vi "Load_from_Project.vi"(8 "error in (no error)":errorcluster, 9 "index":string, 10 "buildObject":T1, 11 "IB_RegData in":refnum<class "IB_RegData.lvclass">) -> (0 "error out":errorcluster, 1 "index out":string, 2 "buildObject out":T1, 3 "IB_RegData out":refnum<class "IB_RegData.lvclass">)   [LabVIEW 2020, in "IB_RegData.lvclass"]
uses:
  <vilib>/AppBuilder/IB_Classes/RegData/IB_RegData.lvclass
  <vilib>/AppBuilder/IB_Classes/RegData/IB_RegData.lvclass/IB_RegData.ctl
  <vilib>/AppBuilder/IB_RW_Project/IB_RW_Project_PropBag_Action.ctl
  <resource>/Framework/Providers/API/ItemRef.ctl
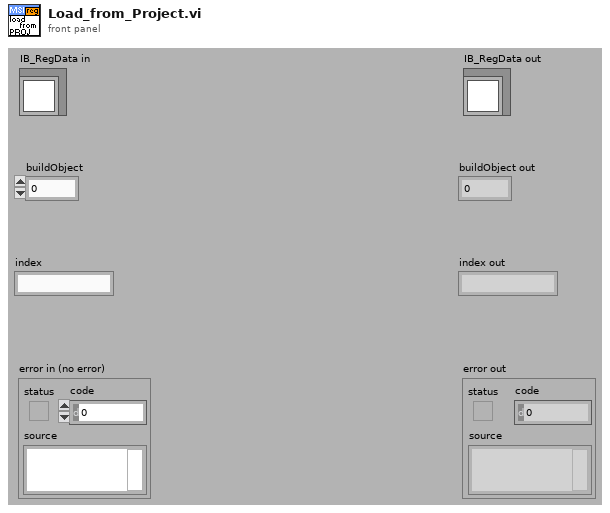
[diagram p1: front panel]
types:
  T1 = typedef "ItemRef.ctl" = u64
  T2 = typedef "IB_RW_Project_PropBag_Action.ctl" = enum16{"read", "write", "clear", "readPrevious", "writePrevious", "clearPrevious"}
  T3 = typedef "IB_RW_Project_RegData_Data.ctl" = cluster{"name":string, "unlock":bool}
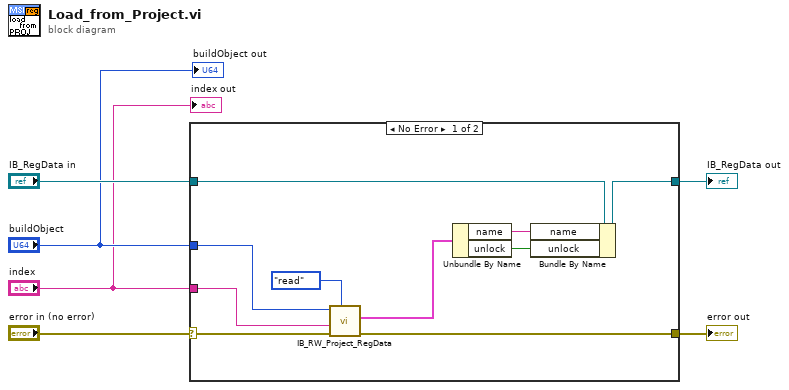
[diagram p0: block diagram]
diagram:
  n1 = case shown="No Error" "error in (no error)" {
    selector: "error in (no error)" -> [w16 w18]
    tunnel: [w15 w18] -> w5
    tunnel: [w10 w17] -> w3
    tunnel: "IB_RegData in" -> [w11 w17]
    tunnel: "buildObject" -> [w14 _]
    tunnel: "index" -> [w12 _]
    frame No Error {
      n2 = call <vilib>:"IB_RW_Project_RegData.vi"("action"=IB_RW_Project_PropBag_Action."read", "error in (no error)"=w16, "index in"=w12, "buildObject"=w14) -> ("error out"=w15:errorcluster, "RegData"=w9:T3)  [unwired: 4 in, 2 out]
      n3 = Unbundle By Name(w9) -> ("name"=w8:string, "unlock"=w7:bool)
      n4 = Bundle By Name(cluster=w11, "name"=w8, "unlock"=w7) -> (w10:refnum<class "IB_RegData.lvclass">)
    }
    frame Error {
    }
  }
  "error out" <- w5
  "IB_RegData out" <- w3
  "buildObject out" <- "buildObject"
  "index out" <- "index"
